vi "Recieve.vi"(8 "error in (no error)":errorcluster, 9 "timeout in ms (-1)":i32=-1, 11 "Get Refnum in":refnum<class "Get Refnum.lvclass">) -> (0 "error out":errorcluster, 1 "Success?":bool, 3 "VI Refnum":refnum<vi>)   [LabVIEW 2020, in "Msg.lvlib" / "Get Refnum.lvclass"]
doc: "Recieve the VI refnum from the queue."
uses:
  Get Refnum.lvclass
  Get Refnum.lvclass/Get Refnum.ctl
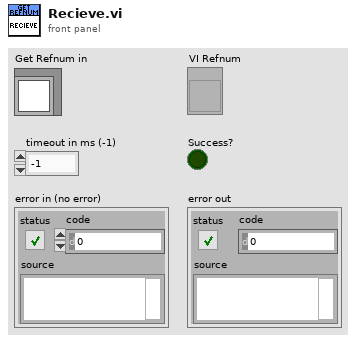
[diagram p1: front panel]
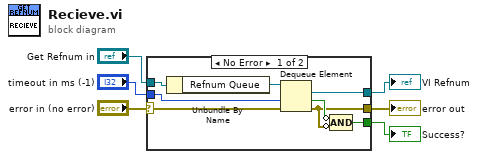
[diagram p0: block diagram]
diagram:
  n1 = case shown="No Error" "error in (no error)" {
    selector: "error in (no error)" -> [w10 w15]
    tunnel: "Get Refnum in" -> [w14 _]
    tunnel: "timeout in ms (-1)" -> [w12 _]
    tunnel: [w11 _] -> w1
    tunnel: [w8 _] -> w3
    tunnel: [w7 w15] -> w2
    frame No Error {
      n2 = Unbundle By Name(w14) -> ("Refnum Queue"=w13:refnum<queue>)
      n3 = Dequeue Element(queue=w13, timeout in ms (-1)=w12, error in (no error)=w10) -> (element=w11:refnum<vi>, timed out?=w9:bool, error out=w7:errorcluster)  [unwired: 1 out]
      n4 = Compound Arithmetic op=AND(invert w9, invert w7) -> (w8:bool)
    }
    frame Error {
    }
  }
  "error out" <- w2
  "Success?" <- w3
  "VI Refnum" <- w1
